vi "xxxx Core.vi"(8 "error in (no error)":errorcluster, 11 "B Context State in":refnum<class "B Context State.lvclass">) -> (0 "error out":errorcluster, 3 "B Context State out":refnum<class "B Context State.lvclass">)   [LabVIEW 2021, in "Context.lvlib" / "B Context State.lvclass"]
uses:
  B Context State.lvclass
  B Context State.lvclass/B Context State.ctl
  Context/Context.lvclass/Context.ctl
  Context/Read Context I32.vi
  Context/Write Context I32.vi
  Context/Context.lvclass
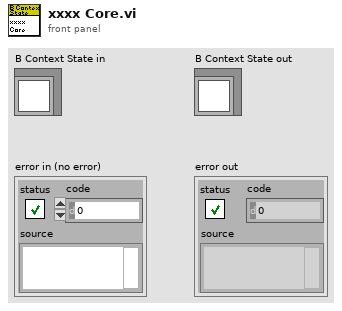
[diagram p1: front panel]
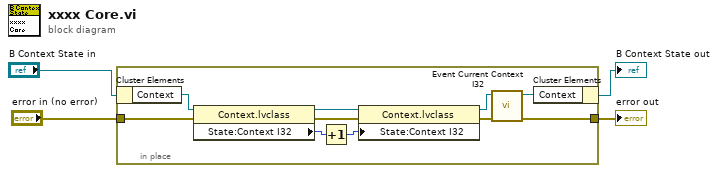
[diagram p0: block diagram]
diagram:
  n1 = in-place {
    in-place-border: "error in (no error)" -> [w10]
    in-place-border: [w5] -> w1
    n2 = in-place-cluster #1("B Context State in") -> ("Context"=w14:refnum<class "Context.lvclass">)
    n3 = property class="Context.lvclass"(reference=w14, error in=w10) -> (reference out=w13:refnum<class "Context.lvclass">, error out=w9:errorcluster, "State:Context I32"=w12:i32)
    n4 = Increment(x=w12) -> (x+1=w11:i32)
    n5 = property class="Context.lvclass"(reference=w13, error in=w9, "State:Context I32"=w11) -> (reference out=w8:refnum<class "Context.lvclass">, error out=w6:errorcluster)
    n6 = call "Event Current Context I32.vi"("error in (no error)"=w6, "Context in"=w8) -> ("error out"=w5:errorcluster, "Context out"=w7:refnum<class "Context.lvclass">)  [unwired: 8 in]
    n7 = in-place-cluster #1("Context"=w7) -> (→"B Context State out":refnum<class "B Context State.lvclass">)
  }
  "error out" <- w1
